vi "VG_OCV70max_P.vi"() -> ()   [LabVIEW 2020]
panel:
  out "OCV70max":dbl
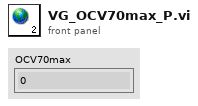
[diagram p1: front panel]
diagram:
